vi "EventLogger.Event.vi"(8 "error in":errorcluster, 9 "Event Description":string, 10 "Event Name":string) -> (0 "error out":errorcluster)   [LabVIEW 2019, in "Tools.lvlib"]
uses:
  Tools.lvlib
  <vilib>/NI/Event Logger Library/EventLog/EventLog.lvclass
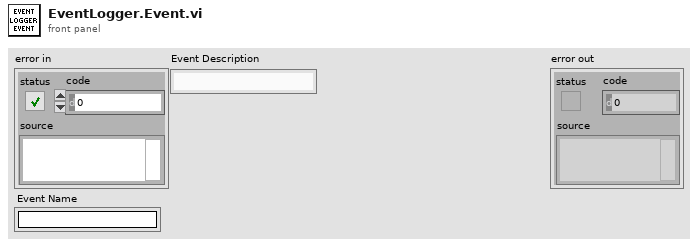
[diagram p1: front panel]
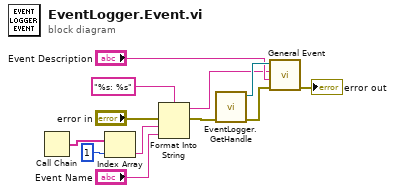
[diagram p0: block diagram]
diagram:
  n1 = Call Chain() -> (call chain=w9:string[])
  n2 = Index Array(array=w9, index=1) -> (element=w7:string)
  n3 = Format Into String(format string="%s: %s", error in="error in", w7, "Event Name") -> (resulting string=w4:string, error out=w2:errorcluster)  [unwired: 1 in]
  n4 = call "EventLogger.GetHandle.vi"("error in"=w2) -> ("error out"=w1:errorcluster, "EventLog ref"=w12:refnum<class "EventLog.lvclass">)  [unwired: 9 in]
  n5 = call <vilib>:"General Event.vi"("error in (no error)"=w1, "Event Description"="Event Description", "Event Name"=w4, "EventLog ref"=w12) -> ("error out"=→"error out":errorcluster)  [unwired: 6 in, 1 out]
